vi "Check Error Status.vi"(8 "error in (no error)":errorcluster, 11 "navX Error Status in":refnum<class "navX Error Status.lvclass">) -> (0 "error out":errorcluster, 2 "Timeout!":bool, 3 "navX Error Status out":refnum<class "navX Error Status.lvclass">)   [LabVIEW 2015, in "navX Library v3.lvlib" / "navX Error Status.lvclass"]
uses:
  navX Error Status.lvclass
  navX Error Status.lvclass/navX Error Status.ctl
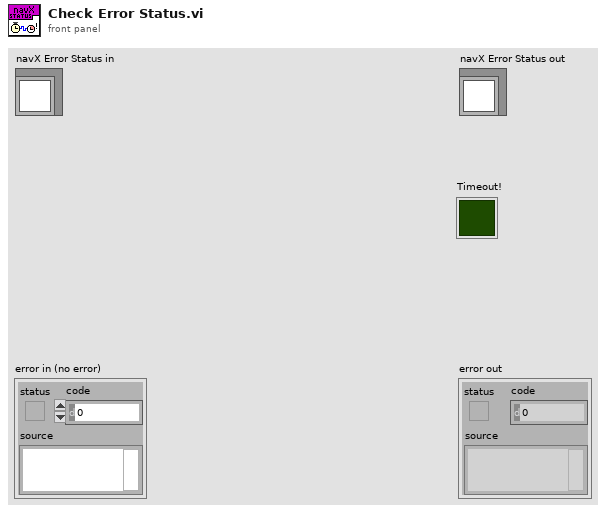
[diagram p1: front panel]
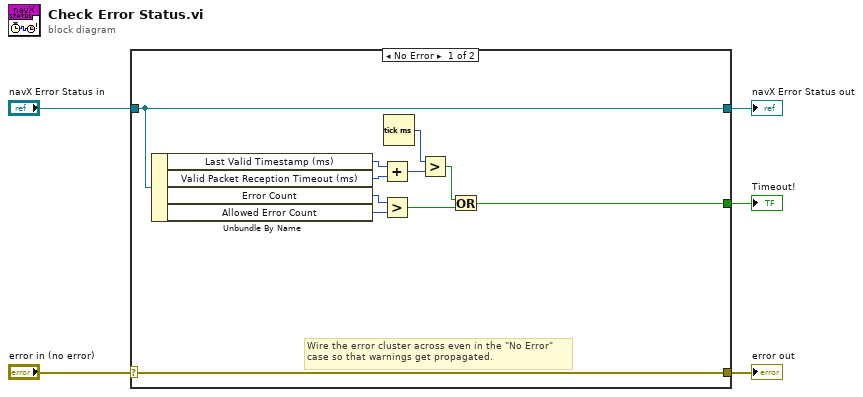
[diagram p0: block diagram]
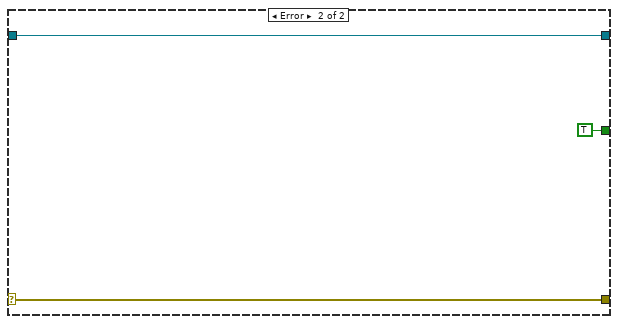
[diagram p2: hidden frame]
diagram:
  n1 = case shown="No Error" "error in (no error)" {
    selector: "error in (no error)" -> [w16 w19]
    tunnel: [w16 w19] -> w4
    tunnel: [w15 w18] -> w2
    tunnel: "navX Error Status in" -> [w15 w18]
    tunnel: [w6 TRUE] -> w1
    frame No Error {
      # "Wire the error cluster across even in the \"No Error\"\ncase so that warnings get propagated."
      n2 = Unbundle By Name(w15) -> ("Last Valid Timestamp (ms)"=w11:u32, "Valid Packet Reception Timeout (ms)"=w12:u32, "Error Count"=w14:i32, "Allowed Error Count"=w13:i32)
      n3 = Add(x=w11, y=w12) -> (x+y=w10:u32)
      n4 = Greater?(x=w14, y=w13) -> (0:w7:bool)
      n5 = Tick Count (ms)() -> (millisecond timer value=w9:u32)
      n6 = Greater?(x=w9, y=w10) -> (0:w8:bool)
      n7 = Or(x=w8, y=w7) -> (x .or. y?=w6:bool)
    }
    frame Error {
    }
  }
  "error out" <- w4
  "navX Error Status out" <- w2
  "Timeout!" <- w1
